vi "Mean_Gamma_Deviance.vi"(8 "error in (no error)":errorcluster caption="entrée d'erreur (pas d'erreur)", 9 "y_pred":string[][](array[string]), 10 "y_true":string[][](array[string]), 11 "mean_gamma_deviance":cluster{"sample_weight":dbl[]}) -> (0 "error out":errorcluster caption="sortie d'erreur", 3 "Score":string)   [LabVIEW 2020]
doc: "Mean Gamma deviance regression loss.\n\nGamma deviance is equivalent to the Tweedie deviance with the power parameter power=2. It is invariant to scaling of the target variable, and measures relative errors.\n\n\n\nParameters : \n\n- y_true : array-like of shape (n_samples,)\nGround truth (correct) target values. Requires y_true > 0.\n\n- y_pred : array-like of shape (n_samples,)\nEstimated target values. Requires y_pred > 0.\n\n- sample_weight : array-like of shape (n_samples,), default=None\nSample weights.\n\nReturns :\n \n- loss : float\nA non-negative floating point value (the best value is 0.0)."
uses:
  Mean_Gamma_Deviance.lvclass
panel:
  out "Mean_Gamma_Deviance.lvclass":refnum<class "Mean_Gamma_Deviance.lvclass">
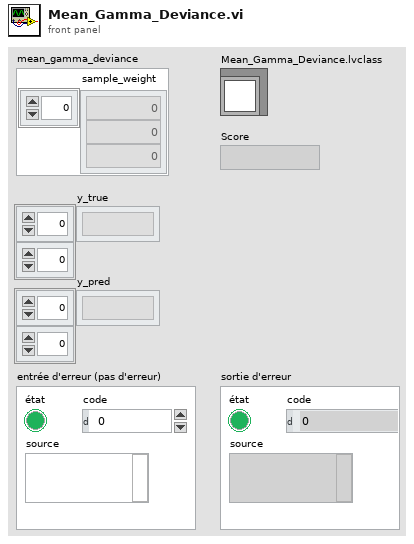
[diagram p1: front panel]
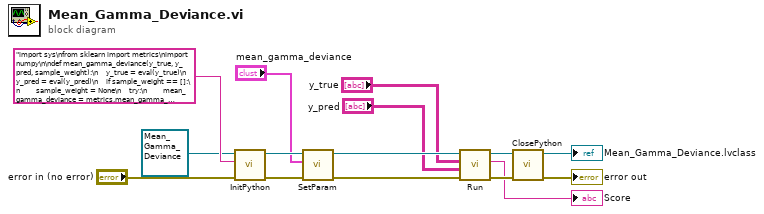
[diagram p0: block diagram]
diagram:
  n1 = call-dynamic "InitPython.vi"("error in (no error)"="error in (no error)", "Python Instruction"="import sys\nfrom sklearn import metrics\nimport numpy\n\ndef mean_gamma_deviance(y_true, y_pred, sample_weight):\n    y_true = eval(y_true)\n    y_pred = eval(y_pred)\n    if sample_weight == []:\n        sample_weight = None\n    try:\n        mean_gamma_deviance = metrics.mean_gamma_deviance(y_true, y_pred, sample_weight)\n        mean_gamma_deviance = mean_gamma_deviance.tolist()\n        return str(mean_gamma_deviance)\n    except:\n        erreur = sys.exc_info()\n        typerr = u\"%s\" % (erreur[0])\n        typerr = typerr[typerr.find(\"'\")+1:typerr.rfind(\"'\")]\n        msgerr = u\"%s\" % (erreur[1])\n        message = str('/!\\\\ {0} : {1}'. format(typerr,msgerr))\n        return message", "Scikit-learn en entrée"=refnum<class "Mean_Gamma_Deviance.lvclass"> refnum ("Mean_Gamma_Deviance.lvclass")) -> ("error out"=w11:errorcluster, "Scikit-learn en sortie"=w10:refnum<class "Mean_Gamma_Deviance.lvclass">)  [unwired: 7 in]
  n2 = call-dynamic "SetParam.vi"("error in (no error)"=w11, "mean_gamma_deviance"="mean_gamma_deviance", "Mean_Gamma_Deviance.lvclass"=w10) -> ("error out"=w7:errorcluster, "Mean_Gamma_Deviance.lvclass"=w8:refnum<class "Mean_Gamma_Deviance.lvclass">)  [unwired: 7 in]
  n3 = call-dynamic "Run.vi"("error in (no error)"=w7, "y_pred"="y_pred", "y_true"="y_true", "Mean_Gamma_Deviance.lvclass"=w8) -> ("error out"=w6:errorcluster, "String Data"=→"Score":string, "Mean_Gamma_Deviance.lvclass"=w5:refnum<class "Mean_Gamma_Deviance.lvclass">)  [unwired: 5 in]
  n4 = call-dynamic "ClosePython.vi"("error in (no error)"=w6, "Scikit-learn en entrée"=w5) -> ("error out"=→"error out":errorcluster, "Scikit-learn en sortie"=→"Mean_Gamma_Deviance.lvclass":refnum<class "Mean_Gamma_Deviance.lvclass">)  [unwired: 8 in]
